vi "MT Rayleigh Fading Profile (Jakes).vi"(0 "profile length (samples)":i32=1000, 5 "sampling frequency (Hz)":dbl=1.0 format="%.2f", 7 "doppler spread (Hz)":dbl=0.01 format="%.2p", 9 "seed in (0xFFFFFFFF)":i32=-1 format="%.0x", 11 "error in (no error)":errorcluster, 12 "fading variance":dbl=1.0 format="%.2f", 13 "reset? (T)":bool=TRUE) -> (4 "fading profile":cdb[](array[numeric]) format="%.2f", 10 "seed out":i32 format="%.0x", 15 "error out":errorcluster)   [LabVIEW 2020, in "niDMT.lvlib"]
doc: "This polymorphic instance generates a Rayleigh flat-fading profile with an envelope that statistically obeys the Rayleigh distribution, using the Jakes fading model."
uses:
  <vilib>/addons/Modulation/niDMT.lvlib
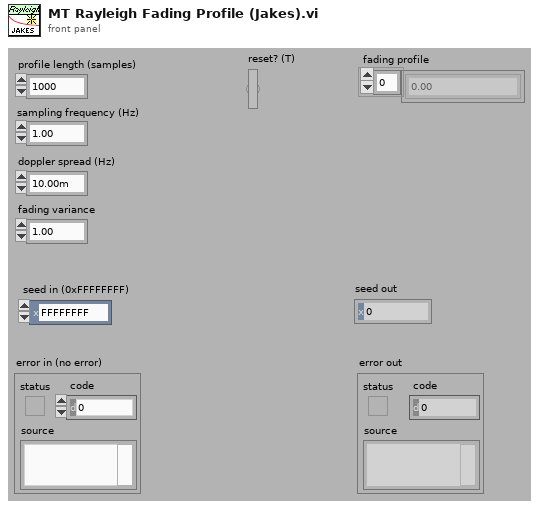
[diagram p1: front panel]
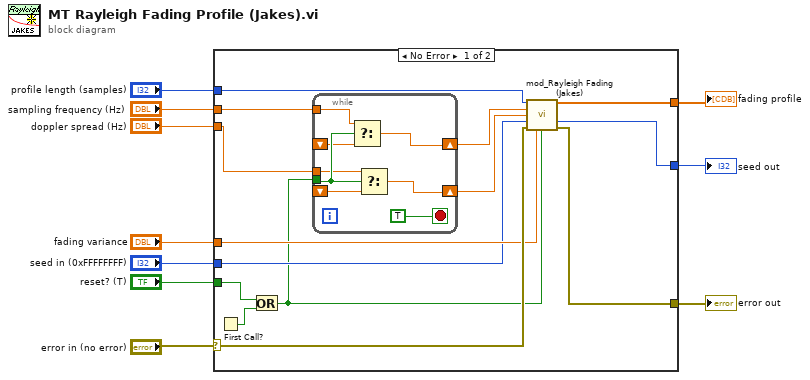
[diagram p0: block diagram]
diagram:
  n1 = case shown="No Error" "error in (no error)" {
    selector: "error in (no error)" -> [w21 w33]
    tunnel: "profile length (samples)" -> [w22 _]
    tunnel: [w24 _] -> w9
    tunnel: [w23 w33] -> w8
    tunnel: "sampling frequency (Hz)" -> [w16 _]
    tunnel: "doppler spread (Hz)" -> [w14 _]
    tunnel: "fading variance" -> [w20 _]
    tunnel: "reset? (T)" -> [w17 _]
    tunnel: "seed in (0xFFFFFFFF)" -> [w18 _]
    tunnel: [w11 _] -> w1
    frame No Error {
      n2 = First Call?() -> (First Call?: T/F=w19:bool)
      n3 = Or(x=w17, y=w19) -> (x .or. y?=w15:bool)
      n4 = while {
        tunnel: w15 -> [w31]
        tunnel: w16 -> [w30]
        shift-right: [w29] -> w13
        shift-left: _ -> [w28]
        tunnel: w14 -> [w27]
        shift-right: [w26] -> w12
        shift-left: _ -> [w25]
        stop <- TRUE stop-if-true
        n5 = Select(t=w30, s=w31, f=w28) -> (s? t:f=w29:dbl)
        n6 = Select(t=w27, s=w31, f=w25) -> (s? t:f=w26:dbl)
      }
      n7 = call <vilib>:"mod_Rayleigh Fading (Jakes).vi"("profile length (samples)"=w22, "sampling frequency (Hz)"=w13, "doppler spread (Hz)"=w12, "seed in (0xFFFFFFFF)"=w18, "error in (no error)"=w21, "fading variance"=w20, "reset? (T)"=w15) -> ("rayleigh fading profile"=w24:cdb[], "next seed"=w11:i32, "error out"=w23:errorcluster)  [unwired: 6 out]
    }
    frame Error {
    }
  }
  "fading profile" <- w9
  "error out" <- w8
  "seed out" <- w1
